vi "Fetch From Buffer (Multiple Points).vi"(6 "Buffer Elements":u16(ring) items=["Date", "Extra", "Formatted", "Fractional", "Relative", "Seconds", "Status", "Time", "Timestamp", "Unit"], 8 "error in (no error)":errorcluster, 9 "Timeout (10000 ms)":i32=10000 format="%#.6g", 10 "Buffer Name":string="defbuffer1", 11 "VISA resource name":refnum<visa-resource-name>) -> (0 "error out":errorcluster, 1 "Element Value":string[](array[string]), 2 "Measurements":dbl[](array[numeric]), 3 "VISA resource name out":refnum<visa-resource-name>)   [LabVIEW 2025, in "Keithley DMM7510.lvlib"]
doc: "Reads and returns multiple measurements from the instrument. Returns specified data elements from a specified reading buffer. This VI does not initiate a trigger."
uses:
  Keithley DMM7510.lvlib
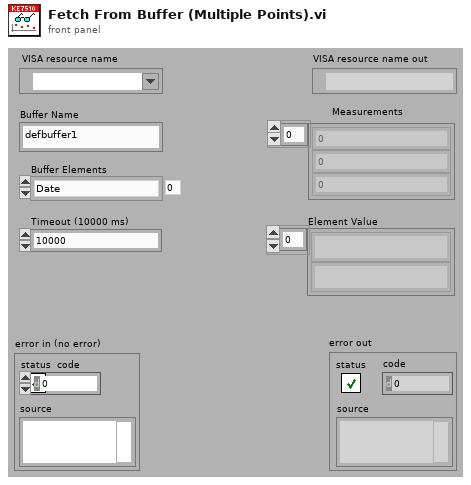
[diagram p1: front panel]
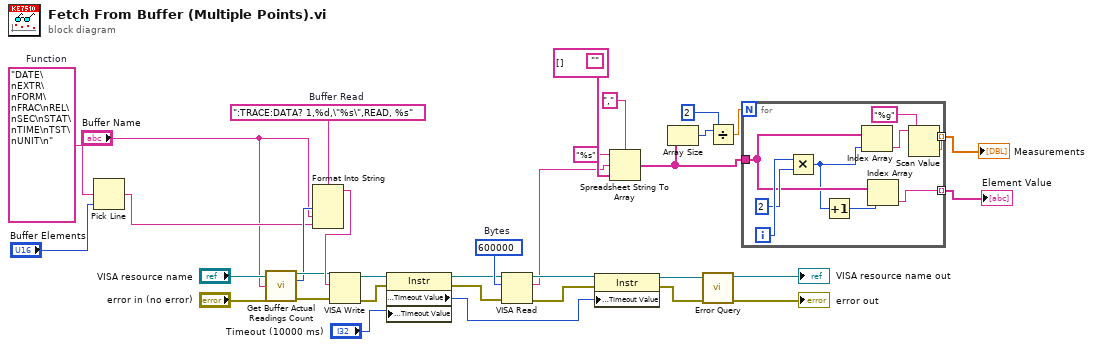
[diagram p0: block diagram]
diagram:
  (unwired) ""
  w18 = "DATE\nEXTR\nFORM\nFRAC\nREL\nSEC\nSTAT\nTIME\nTST\nUNIT\n"  # Function
  w21 = ":TRACE:DATA? 1,%d,\"%s\",READ, %s"  # Buffer Read
  w34 = u32 600000  # Bytes
  n1 = Pick Line(multi-line string=w18, line index="Buffer Elements") -> (output string=w2:string)  [unwired: 1 out]
  n2 = call "Get Buffer Actual Readings Count.vi"("VISA resource name"="VISA resource name", "Buffer Name (defbuffer1)"="Buffer Name", "error in (no error)"="error in (no error)") -> ("VISA resource name out"=w4:refnum<visa-resource-name>, "Actual Readings"=w3:i32, "error out"=w5:errorcluster)  [unwired: 10 in]
  n3 = Format Into String(format string=w21, w3, "Buffer Name", w2) -> (resulting string=w20:string)  [unwired: 2 in, 1 out]
  n4 = VISA Write(VISA resource name=w4, write buffer=w20, error in (no error)=w5) -> (VISA resource name out=w31:refnum<visa-resource-name>, error out=w30:errorcluster)  [unwired: 1 out]
  n5 = property class="Instr"(reference=w31, error in=w30, "General Settings:Timeout Value"="Timeout (10000 ms)") -> (reference out=w29:refnum<visa-resource-name>, error out=w28:errorcluster, "General Settings:Timeout Value"=w22:u32)
  n6 = VISA Read(VISA resource name=w29, byte count=w34, error in (no error)=w28) -> (VISA resource name out=w26:refnum<visa-resource-name>, read buffer=w8:string, error out=w24:errorcluster)  [unwired: 1 out]
  n7 = property class="Instr"(reference=w26, error in=w24, "General Settings:Timeout Value"=w22) -> (reference out=w25:refnum<visa-resource-name>, error out=w23:errorcluster)
  n8 = Spreadsheet String To Array(delimiter (Tab)=",", format string="%s", spreadsheet string=w8, array type (2D Dbl)=string[] []) -> (array=w15:string[])
  n9 = Array Size(array=w15) -> (size(s)=w13:i32)
  n10 = call "Error Query.vi"("error in (no error)"=w23, "VISA resource name"=w25) -> ("error out"=→"error out":errorcluster, "VISA resource name out"=→"VISA resource name out":refnum<visa-resource-name>)  [unwired: 6 in, 2 out]
  n11 = Divide(x=w13, y=2) -> (x/y=w11:dbl)
  n12 = for {
    N: w11 -> [_]
    tunnel: w15 -> [w41]
    tunnel: [w36] -> w10 mode=indexing
    tunnel: [w39] -> w9 mode=indexing
    i -> [w43]
    n13 = Multiply(x=w43, y=2) -> (x*y=w35:i32)
    n14 = Increment(x=w35) -> (x+1=w40:i32)
    n15 = Index Array(array=w41, index=w35) -> (element=w38:string)
    n16 = Index Array(array=w41, index=w40) -> (element=w39:string)
    n17 = Scan Value(string=w38, format string="%g") -> (value=w36:dbl)  [unwired: 1 in, 1 out]
  }
  "Measurements" <- w10
  "Element Value" <- w9
